vi "Generate Action from string.vi"(8 "Error In":errorcluster, 11 "Command Text":string) -> (0 "Error Out":errorcluster, 3 "Action":T1)   [LabVIEW 2012]
uses:
  Custom Controls and Typedefs/Macro_Action_List.ctl
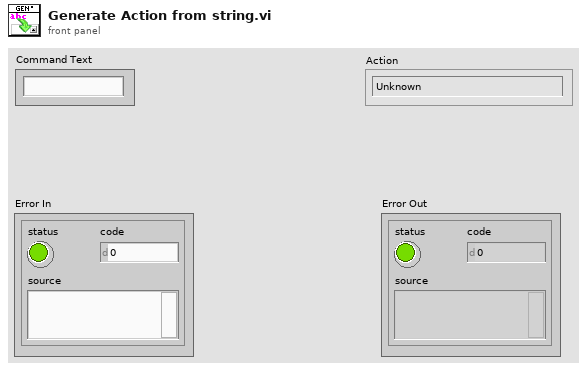
[diagram p1: front panel]
types:
  T1 = typedef "Macro_Action_List.ctl" = enum16{"Unknown", "2D.Frame.Scan", "2D.Line.Scan", "Load.Settings.File", "Move.To.Position", "Pause", "Z.Stack", "LOOP.Start", "LOOP.End"}
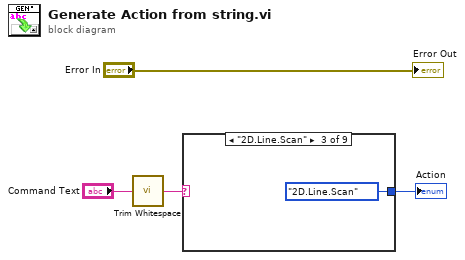
[diagram p0: block diagram]
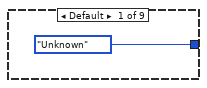
[diagram p2: hidden frame]
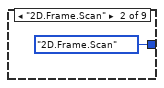
[diagram p3: hidden frame]
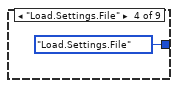
[diagram p4: hidden frame]
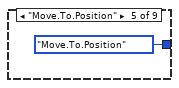
[diagram p5: hidden frame]
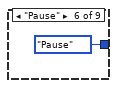
[diagram p6: hidden frame]
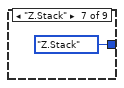
[diagram p7: hidden frame]
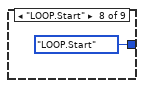
[diagram p8: hidden frame]
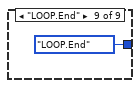
[diagram p9: hidden frame]
diagram:
  n1 = call <vilib>:"Trim Whitespace.vi"("string"="Command Text") -> ("trimmed string"=w2:string)  [unwired: 1 in]
  n2 = case shown="\"2D.Line.Scan\"" w2 {
    tunnel: [Macro_Action_List."Unknown" ("Action") Macro_Action_List."2D.Frame.Scan" ("Action") Macro_Action_List."2D.Line.Scan" ("Action") Macro_Action_List."Load.Settings.File" ("Action") Macro_Action_List."Move.To.Position" ("Action") Macro_Action_List."Pause" ("Action") Macro_Action_List."Z.Stack" ("Action") Macro_Action_List."LOOP.Start" ("Action") Macro_Action_List."LOOP.End" ("Action")] -> w3
    frame Default {
    }
    frame "2D.Frame.Scan" {
    }
    frame "2D.Line.Scan" {
    }
    frame "Load.Settings.File" {
    }
    frame "Move.To.Position" {
    }
    frame "Pause" {
    }
    frame "Z.Stack" {
    }
    frame "LOOP.Start" {
    }
    frame "LOOP.End" {
    }
  }
  "Action" <- w3
  "Error Out" <- "Error In"
